vi "returnSameString.vi"(1 "String":string="\u0017èÿÿ\u0000\u0000`@\u0000\u0000HD\u0000\u0000úC\u0000\u0000HB¤\u0005•") -> (0 "substring":string)   [LabVIEW 2017]
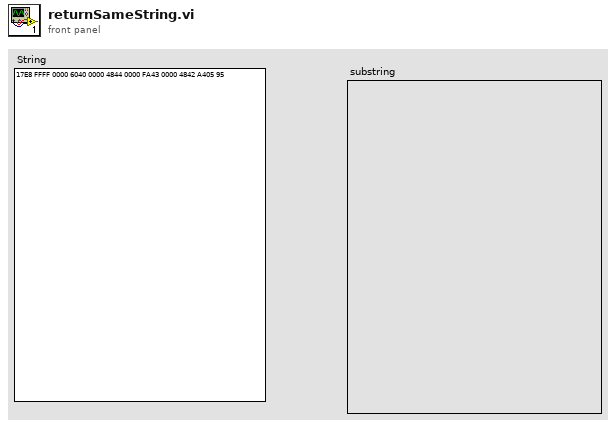
[diagram p1: front panel]
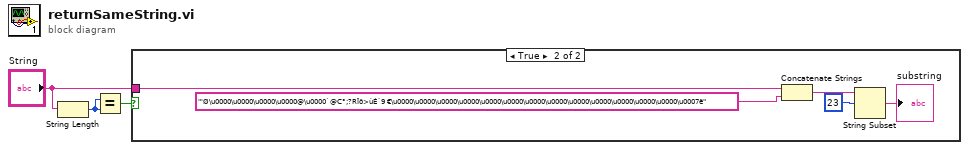
[diagram p0: block diagram]
diagram:
  n1 = String Length(string="String") -> (length=w2:i32)
  n2 = Equal?(x=w2, y=w2) -> (x = y?=w1:bool)
  n3 = case shown="True" w1 {
    tunnel: "String" -> [_ w8]
    frame False {
    }
    frame True {
      n4 = Concatenate Strings(w8, "'Ø\u0000\u0000\u0000\u0000@\u0000`@C°;?RÏð>ùÉ´9 €\u0000\u0000\u0000\u0000\u0000\u0000\u0000\u0000\u0000\u0000\u0000\u0000\u0000\u0007ë" ("string")) -> (w6:string)
      n5 = String Subset(string=w6, offset (0)=23) -> (substring=→"substring":string)  [unwired: 1 in]
    }
  }
